vi "Teleop.vi"(10 "Match Info":T1={"Autonomous Elapsed Seconds"=0.0, "TeleOp Elapsed Seconds"=0.0, "Disabled Elapsed Seconds"=0.0, "Visited Autonomous"=FALSE, "Visited TeleOp"=FALSE, "Visited Disabled"=FALSE, "Autonomous Settings"={"Autonomous Style"=enum."Independent", "VI Refnum"=refnum}}, 11 "Call Context":T2) -> ()   [LabVIEW 2015]
doc: "This VI is called for each TeleOp packet received from the DS where the robot is not disabled. It is often used to read from the joysticks and update I/O or to update setpoints for timed control loops. It should complete and return within 20 milliseconds or it may miss DS packets."
uses:
  <vilib>/Rock Robotics/WPI/DriverStation/WPI_DriverStationDerivedRobotMode.ctl
  <vilib>/Rock Robotics/WPI/DriverStation/WPI_DriverStationMatch Info.ctl
  <vilib>/Rock Robotics/WPI/Solenoid/WPI_SolenoidValue.ctl
  <vilib>/Rock Robotics/WPI/Utilities/WPI_GetSetVariantRefNum.vi
  <vilib>/Rock Robotics/Network Tables/NT Read Boolean.vi
  <vilib>/Rock Robotics/Network Tables/NT Read Number.vi
  <vilib>/Rock Robotics/WPI/Solenoid/WPI_SolenoidSetEnum.vi
panel:
  out "Encodeur gauche max":dbl
  out "Encodeur droit max":dbl
  out "Encodeur gauche min":dbl
  out "Encodeur droit min":dbl
  out "Encodeur gauche":dbl
  out "Encodeur droit":dbl
  out "Sample Slider 0":dbl(slide) scale=0.0..5.0
  out "Sample Boolean 1":bool
  out "Sample Boolean 0":bool
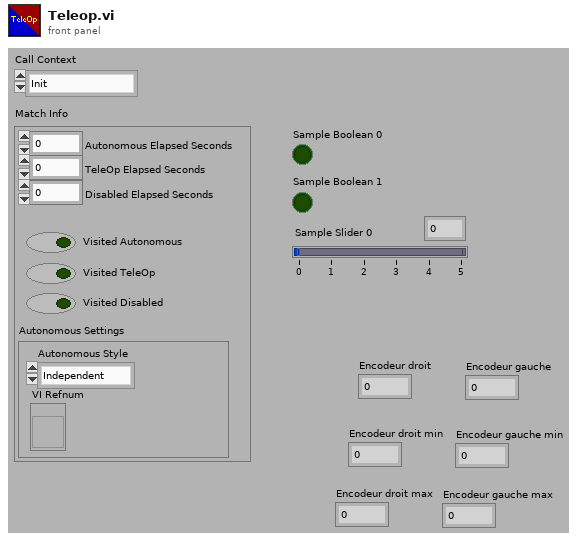
[diagram p1: front panel]
types:
  T1 = typedef "WPI_DriverStationMatch Info.ctl" = cluster{"Autonomous Elapsed Seconds":dbl, "TeleOp Elapsed Seconds":dbl, "Disabled Elapsed Seconds":dbl, "Visited Autonomous":bool, "Visited TeleOp":bool, "Visited Disabled":bool, "Autonomous Settings":cluster{"Autonomous Style":enum16{"Iterative", "Independent"}, "VI Refnum":refnum<vi>}}
  T2 = typedef "WPI_DriverStationDerivedRobotMode.ctl" = enum16{"Init", "Execute", "Stop"}
  T3 = typedef "WPI_SolenoidValue.ctl" = enum16{"Off", "On", "Forward", "Reverse"}
  T4 = typedef "WPI_SolenoidDevRef.ctl" = cluster{"DevStatus":errorcluster, "Pneumatics Control Module":u8, "Forward Solenoid Channel":T5, "Reverse Solenoid Channel":T5}
  T5 = typedef "WPI_SolenoidChannel.ctl" = enum8{"Solenoid 0", "Solenoid 1", "Solenoid 2", "Solenoid 3", "Solenoid 4", "Solenoid 5", "Solenoid 6", "Solenoid 7", "Invalid"}
  T6 = typedef "WPI_JoystickDevRef.ctl" = cluster{"Device":T7}
  T7 = typedef "WPI_JoystickDeviceEnum.ctl" = enum16{"USB 0", "USB 1", "USB 2", "USB 3", "USB 4", "USB 5"}
  T8 = cluster{"Buttons[0]":bool, "Buttons[1]":bool, "Buttons[2]":bool, "Buttons[3]":bool, "Buttons[4]":bool, "Buttons[5]":bool, "Buttons[6]":bool, "Buttons[7]":bool, "Buttons[8]":bool}
  T9 = cluster{"Axes[0]":dbl, "Axes[1]":dbl, "Axes[2]":dbl, "Axes[3]":dbl, "Axes[4]":dbl, "Axes[5]":dbl, "Axes[6]":dbl, "Axes[7]":dbl, "Axes[8]":dbl}
  T10 = typedef "WPI_RobotDriveDevRef.ctl" = cluster{"DevStatus":errorcluster, "Motors[]":T11[], "Square Inputs":bool, "Max Output":dbl}
  T11 = typedef "WPI_MotorControlDeviceRef.ctl" = cluster{"DeviceStatus":errorcluster, "Type":T12, "PWM":cluster{"PWM Channel":T13, "DeadBand":T14}, "CAN":cluster{"Device Number":u8, "Control Mode":T15, "Semaphore":T16, "Max Vout":dbl, "TalonSRX Control Mode":T17}, "Invert":bool}
  T12 = typedef "WPI_MotorControlType.ctl" = enum16{"PWM", "CAN", "CANTalonSRX"}
  T13 = typedef "FPGA_DIOPWMChannel.ctl" = enum8{"PWM 0", "PWM 1", "PWM 2", "PWM 3", "PWM 4", "PWM 5", "PWM 6", "PWM 7", "PWM 8", "PWM 9", "PWM MXP 0", "PWM MXP 1", "PWM MXP 2", "PWM MXP 3", "PWM MXP 4", "PWM MXP 5", "PWM MXP 6", "PWM MXP 7", "PWM MXP 8", "PWM MXP 9", "Invalid"}
  T14 = typedef "WPI_PWMDeadband.ctl" = cluster{"Name":string, "maxPositivePwm":i32, "minPositivePwm":i32, "centerPwm":i32, "maxNegativePwm":i32, "minNegativePwm":i32, "angularRange":u16}
  T15 = typedef "WPI_CANJaguar_ControlMode.ctl" = enum8{"Percent VBus", "Current", "Speed", "Position", "Voltage"}
  T16 = typedef "Semaphore RefNum" = refnum<k1>
  T17 = typedef "WPI_CANTalonSRX_APIControlMode.ctl" = enum8{"Percent VBus", "Speed", "Position", "Slave", "Unchanged / Invalid", "Voltage Compensation", "Current", "Motion Profile"}
  T18 = typedef "WPI_ServoDeviceRef.ctl" = cluster{"DeviceStatus":errorcluster, "PWM Channel":T13, "DeadBand":T14}
  T19 = typedef "WPI_EncoderDevRef.ctl" = cluster{"DevStatus":errorcluster, "EncoderIndex":T20, "CounterIndex":T21, "DistancePerCount":dbl, "Decoding Type":T22}
  T20 = typedef "FPGA_EncoderIdx.ctl" = enum8{"Enc 0", "Enc 1", "Enc 2", "Enc 3", "Enc 4", "Enc 5", "Enc 6", "Enc 7", "Invalid"}
  T21 = typedef "FPGA_CounterCtrSystemIndex.ctl" = enum8{"Ctr 0", "Ctr 1", "Ctr 2", "Ctr 3", "Ctr 4", "Ctr 5", "Ctr 6", "Ctr 7", "Invalid"}
  T22 = typedef "WPI_EncoderType.ctl" = enum16{"1x", "2x", "4x"}
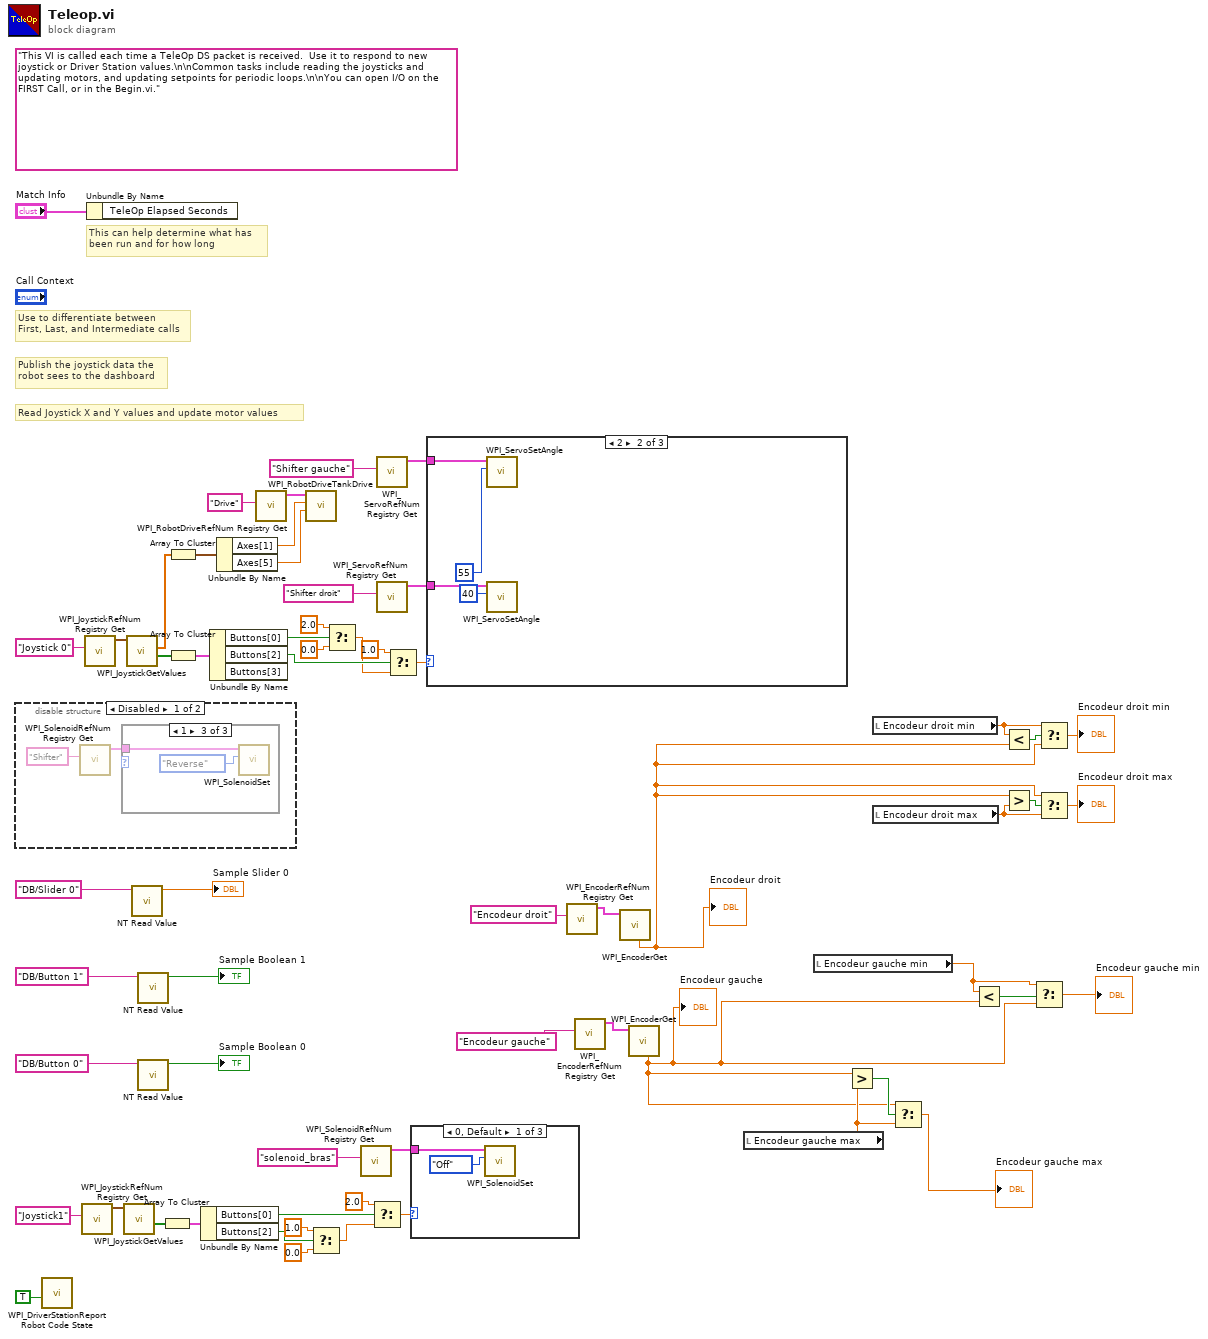
[diagram p0: block diagram]
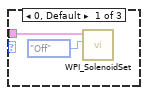
[diagram p2: hidden frame]
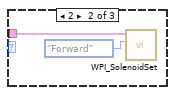
[diagram p3: hidden frame]
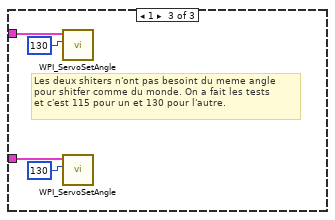
[diagram p6: hidden frame]
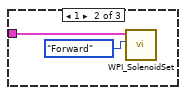
[diagram p7: hidden frame]
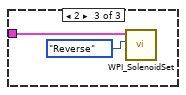
[diagram p8: hidden frame]
diagram:
  (unwired) "This VI is called each time a TeleOp DS packet is received.  Use it to respond to new joystick or Driver Station values.\n\nCommon tasks include reading the joysticks and updating motors, and updating setpoints for periodic loops.\n\nYou can open I/O on the FIRST Call, or in the Begin.vi."
  # "Publish the joystick data the\nrobot sees to the dashboard"
  # "Use to differentiate between\nFirst, Last, and Intermediate calls"
  # "This can help determine what has\nbeen run and for how long"
  # "Read Joystick X and Y values and update motor values"
  n1 = disable-structure shown="Disabled" {
    frame Disabled {
      n2 = call <vilib>:"WPI_SolenoidRefNum Registry Get.vi"("refnum name"="Shifter") -> ("SolenoidDevRef"=w62:T4)  [unwired: 9 in, 1 out]
      n3 = case shown="1" {
        selector: _ -> [_ _ _]
        tunnel: w62 -> [w64 w66 w67]
        frame 0, Default {
          n4 = call-poly <vilib>:"WPI_SolenoidSet.vi"("Value"=WPI_SolenoidValue."Off", "SolenoidDevRef"=w64) -> ()  [unwired: 8 in, 2 out]
        }
        frame 2 {
          n5 = call-poly <vilib>:"WPI_SolenoidSet.vi"("Value"=WPI_SolenoidValue."Forward", "SolenoidDevRef"=w66) -> ()  [unwired: 8 in, 2 out]
        }
        frame 1 {
          n6 = call-poly <vilib>:"WPI_SolenoidSet.vi"("Value"=WPI_SolenoidValue."Reverse", "SolenoidDevRef"=w67) -> ()  [unwired: 8 in, 2 out]
        }
      }
    }
    frame Enabled {
    }
  }
  n7 = call <vilib>:"WPI_DriverStationReport Robot Code State.vi"("TeleOp"=TRUE ("Autonomous")) -> ()  [unwired: 10 in, 1 out]
  n8 = call <vilib>:"WPI_JoystickRefNum Registry Get.vi"("refnum name"="Joystick1") -> ("JoystickDevRef"=w37:T6)  [unwired: 1 in, 9 out]
  n9 = call <vilib>:"WPI_JoystickRefNum Registry Get.vi"("refnum name"="Joystick 0") -> ("JoystickDevRef"=w58:T6)  [unwired: 1 in, 9 out]
  n10 = Unbundle By Name("Match Info") -> ()  [unwired: 1 out]
  n11 = call <vilib>:"WPI_JoystickGetValues.vi"("JoystickDevRef"=w37) -> ("Buttons"=w38:bool[])  [unwired: 6 in, 4 out]
  n12 = call <vilib>:"WPI_JoystickGetValues.vi"("JoystickDevRef"=w58) -> ("Buttons"=w48:bool[], "Axes"=w50:dbl[])  [unwired: 6 in, 3 out]
  n13 = call-poly <vilib>:"NT Read Value.vi"("Name"="DB/Slider 0" ("refnum name")) -> ("Numeric"=→"Sample Slider 0":dbl)  [unwired: 9 in, 1 out]
  n14 = call-poly <vilib>:"NT Read Value.vi"("Name"="DB/Button 1" ("refnum name")) -> ("Boolean"=→"Sample Boolean 1":bool)  [unwired: 9 in, 1 out]
  n15 = call-poly <vilib>:"NT Read Value.vi"("Name"="DB/Button 0" ("refnum name")) -> ("Boolean"=→"Sample Boolean 0":bool)  [unwired: 9 in, 1 out]
  n16 = Array To Cluster(array=w38) -> (cluster=w39:T8)
  n17 = Array To Cluster(array=w50) -> (cluster=w49:T9)
  n18 = Array To Cluster(array=w48) -> (cluster=w47:T8)
  n19 = Unbundle By Name(w39) -> ("Buttons[0]"=w32:bool, "Buttons[2]"=w31:bool)
  n20 = Unbundle By Name(w47) -> ("Buttons[0]"=w46:bool, "Buttons[2]"=w43:bool)  [unwired: 1 out]
  n21 = Unbundle By Name(w49) -> ("Axes[1]"=w25:dbl, "Axes[5]"=w24:dbl)
  n22 = call <vilib>:"WPI_RobotDriveRefNum Registry Get.vi"("refnum name"="Drive") -> ("RobotDriveDevRef"=w51:T10)  [unwired: 9 in, 1 out]
  n23 = call <vilib>:"WPI_RobotDriveTankDrive.vi"("Right axis value"=w24, "Left axis value"=w25, "RobotDriveDevRef"=w51) -> ()  [unwired: 6 in, 3 out]
  n24 = Select(t=1.0, s=w31, f=0.0) -> (s? t:f=w33:dbl)
  n25 = Select(t=2.0, s=w46, f=0.0) -> (s? t:f=w42:dbl)
  n26 = call <vilib>:"WPI_SolenoidRefNum Registry Get.vi"("refnum name"="solenoid_bras") -> ("SolenoidDevRef"=w26:T4)  [unwired: 9 in, 1 out]
  n27 = Select(t=2.0, s=w32, f=w33) -> (s? t:f=w27:dbl)
  n28 = call <vilib>:"WPI_ServoRefNum Registry Get.vi"("refnum name"="Shifter gauche") -> ("ServoDeviceRef"=w20:T18)  [unwired: 9 in, 1 out]
  n29 = call <vilib>:"WPI_ServoRefNum Registry Get.vi"("refnum name"="Shifter droit") -> ("ServoDeviceRef"=w21:T18)  [unwired: 9 in, 1 out]
  n30 = Select(t=1.0, s=w43, f=w42) -> (s? t:f=w19:dbl)
  n31 = case shown="0, Default" w27 {
    tunnel: w26 -> [w69 w72 w73]
    frame 0, Default {
      n32 = call-poly <vilib>:"WPI_SolenoidSet.vi"("Value"=WPI_SolenoidValue."Off", "SolenoidDevRef"=w69) -> ()  [unwired: 8 in, 2 out]
    }
    frame 1 {
      n33 = call-poly <vilib>:"WPI_SolenoidSet.vi"("Value"=WPI_SolenoidValue."Forward", "SolenoidDevRef"=w72) -> ()  [unwired: 8 in, 2 out]
    }
    frame 2 {
      n34 = call-poly <vilib>:"WPI_SolenoidSet.vi"("Value"=WPI_SolenoidValue."Reverse", "SolenoidDevRef"=w73) -> ()  [unwired: 8 in, 2 out]
    }
  }
  n35 = case shown="2" w19 {
    tunnel: w20 -> [_ w78 w82]
    tunnel: w21 -> [_ w77 w81]
    frame 0, Default {
    }
    frame 2 {
      n36 = call <vilib>:"WPI_ServoSetAngle.vi"("Angle"=55, "ServoDeviceRef"=w78) -> ()  [unwired: 8 in, 2 out]
      n37 = call <vilib>:"WPI_ServoSetAngle.vi"("Angle"=40, "ServoDeviceRef"=w77) -> ()  [unwired: 8 in, 2 out]
    }
    frame 1 {
      # "Les deux shiters n'ont pas besoint du meme angle \npour shitfer comme du monde. On a fait les tests \net c'est 115 pour un et 130 pour l'autre."
      n38 = call <vilib>:"WPI_ServoSetAngle.vi"("Angle"=130, "ServoDeviceRef"=w82) -> ()  [unwired: 8 in, 2 out]
      n39 = call <vilib>:"WPI_ServoSetAngle.vi"("Angle"=130, "ServoDeviceRef"=w81) -> ()  [unwired: 8 in, 2 out]
    }
  }
  n40 = call <vilib>:"WPI_EncoderRefNum Registry Get.vi"("refnum name"="Encodeur droit") -> ("EncoderDevRef"=w17:T19)  [unwired: 9 in, 1 out]
  n41 = call <vilib>:"WPI_EncoderRefNum Registry Get.vi"("refnum name"="Encodeur gauche") -> ("EncoderDevRef"=w16:T19)  [unwired: 9 in, 1 out]
  n42 = call <vilib>:"WPI_EncoderGet.vi"("EncoderDevRef"=w17) -> ("Rate"=w1:dbl)  [unwired: 5 in, 5 out]
  "Encodeur droit" <- w1
  n43 = call <vilib>:"WPI_EncoderGet.vi"("EncoderDevRef"=w16) -> ("Rate"=w9:dbl)  [unwired: 5 in, 5 out]
  "Encodeur gauche" <- w9
  n44 = local read "Encodeur gauche max"() -> (w13:dbl)
  n45 = local read "Encodeur gauche min"() -> (w10:dbl)
  n46 = Greater?(x=w9, y=w13) -> (0:w14:bool)
  n47 = local read "Encodeur droit min"() -> (w4:dbl)
  n48 = local read "Encodeur droit max"() -> (w6:dbl)
  n49 = Select(t=w9, s=w14, f=w13) -> (s? t:f=→"Encodeur gauche max":dbl)
  n50 = Less?(x=w10, y=w9) -> (x < y?=w11:bool)
  n51 = Less?(x=w4, y=w1) -> (x < y?=w5:bool)
  n52 = Greater?(x=w1, y=w6) -> (0:w7:bool)
  n53 = Select(t=w10, s=w11, f=w9) -> (s? t:f=→"Encodeur gauche min":dbl)
  n54 = Select(t=w4, s=w5, f=w1) -> (s? t:f=→"Encodeur droit min":dbl)
  n55 = Select(t=w1, s=w7, f=w6) -> (s? t:f=→"Encodeur droit max":dbl)
